vi "CallNode_Create.vi"(0 "reference":refnum<class "CallNode.lvclass">, 5 "error in (no error)":errorcluster) -> (14 "reference out":refnum<class "CallNode.lvclass">, 19 "error out":errorcluster)   [LabVIEW 2014, in "CallNode.lvclass"]
doc: "Creates and initializes a new CallNode object.\n\nThis object should be destroyed using a CallNode destructor VI or a virtual base class destructor VI.\n\n[GOOP 2.3]"
uses:
  <resource>/Framework/Providers/Open_GDS/UML/CallNode_class/CallNode.lvclass
  <resource>/Framework/Providers/Open_GDS/UML/General/Rectangle/Rectangle Rectangle2D.ctl
  <resource>/Framework/Providers/Open_GDS/UML/RectangularNode_class/RectangularNode.lvclass
panel:
  # "The input reference should only\nbe wired when this method is called\nby a sub class constructor."
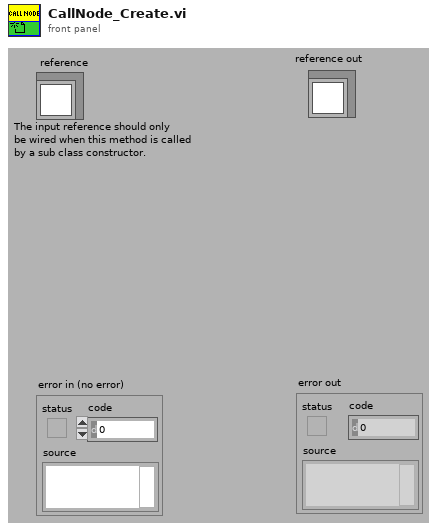
[diagram p1: front panel]
types:
  T1 = typedef "Rectangle Rectangle2D.ctl" = cluster{"x":dbl, "y":dbl, "width":dbl, "height":dbl}
  T2 = typedef "CallNode.lvclass/ClassAttributes.ctl" = cluster{"Base class":T3, "CALL_YGAP":i32}
  T3 = typedef "RectangularNode.lvclass/ClassAttributes.ctl" = cluster{"Base class":T4, "childClassAttribute2":enum16{"Hello", "Goodbye"}}
  T4 = typedef "AbstractNode.lvclass/ClassAttributes.ctl" = cluster{"classAttribute1":bool}
  T5 = typedef "CallNode.lvclass/ObjectAttributes.ctl" = cluster{"objectCallNodeRef":refnum<class "AbstractNode.lvclass">, "signaled":bool, "openBottom":bool, "DEFAULT_WIDTH":i32, "DEFAULT_HEIGHT":i32, "CALL_YGAP":i32}
  T6 = typedef "RectangularNode.lvclass/ObjectAttributes.ctl" = cluster{"bounds":T1}
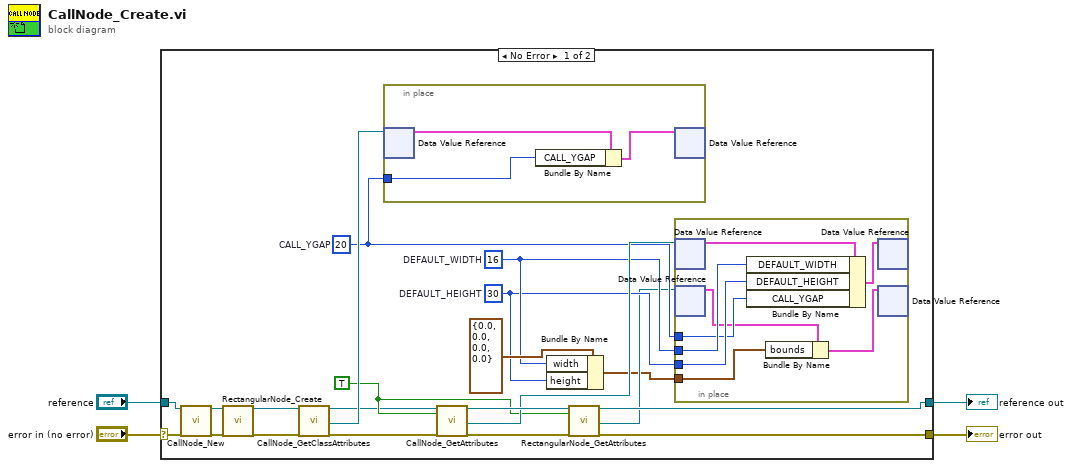
[diagram p0: block diagram]
diagram:
  n1 = case shown="No Error" "error in (no error)" {
    selector: "error in (no error)" -> [w25 w38]
    tunnel: [w12 w37] -> w4
    tunnel: [w5 w38] -> w3
    tunnel: "reference" -> [w24 w37]
    frame No Error {
      w10 = TRUE ("OnlyGetDvrReference(False)")
      w13 = 20  # CALL_YGAP
      w14 = 30  # DEFAULT_HEIGHT
      w15 = 16  # DEFAULT_WIDTH
      n2 = call <resource>:"CallNode_New.vi"("reference in"=w24, "error in (no error)"=w25) -> ("reference out"=w22:refnum<class "CallNode.lvclass">, "error out"=w23:errorcluster)  [unwired: 2 in, 14 out]
      n3 = call <resource>:"RectangularNode_Create.vi"("reference"=w22, "error in (no error)"=w23) -> ("reference out"=w19:refnum<class "CallNode.lvclass">, "error out"=w18:errorcluster)  [unwired: 1 in, 15 out]
      n4 = call <resource>:"CallNode_GetClassAttributes.vi"("reference in"=w19, "error in (no error)"=w18) -> ("reference out"=w6:refnum<class "CallNode.lvclass">, "Class attribute Reference"=w17:refnum<data-value>, "error out"=w7:errorcluster)  [unwired: 14 in, 1 out]
      n5 = in-place {
        in-place-border: w13 -> [w35]
        n6 = in-place-dvr #1(w17) -> (w36:T2)  [unwired: 1 out]
        n7 = Bundle By Name(cluster=w36, "CALL_YGAP"=w35) -> (w34:T2)
        n8 = in-place-dvr #1(w34) -> ()  [unwired: 2 out]
      }
      n9 = call <resource>:"CallNode_GetAttributes.vi"("reference in"=w6, "OnlyGetDvrReference(False)"=w10, "error in (no error)"=w7) -> ("reference out"=w21:refnum<class "CallNode.lvclass">, "DataRef"=w16:refnum<data-value>, "error out"=w11:errorcluster)  [unwired: 13 in, 1 out]
      n10 = Bundle By Name(cluster=T1 {"x"=0.0, "y"=0.0, "width"=0.0, "height"=0.0} ("Base class.bounds"), "width"=w15, "height"=w14) -> (w8:T1)
      n11 = call <resource>:"RectangularNode_GetAttributes.vi"("reference in"=w21, "OnlyGetDvrReference(False)"=w10, "error in (no error)"=w11) -> ("reference out"=w12:refnum<class "CallNode.lvclass">, "DataRef"=w9:refnum<data-value>, "error out"=w5:errorcluster)  [unwired: 13 in, 1 out]
      n12 = in-place {
        in-place-border: w15 -> [w32]
        in-place-border: w14 -> [w31]
        in-place-border: w13 -> [w30]
        in-place-border: w8 -> [w27]
        n13 = in-place-dvr #2(w16) -> (w33:T5)  [unwired: 1 out]
        n14 = in-place-dvr #3(w9) -> (w28:T6)  [unwired: 1 out]
        n15 = Bundle By Name(cluster=w33, "DEFAULT_WIDTH"=w32, "DEFAULT_HEIGHT"=w31, "CALL_YGAP"=w30) -> (w29:T5)
        n16 = Bundle By Name(cluster=w28, "bounds"=w27) -> (w26:T6)
        n17 = in-place-dvr #2(w29) -> ()  [unwired: 2 out]
        n18 = in-place-dvr #3(w26) -> ()  [unwired: 2 out]
      }
    }
    frame Error {
    }
  }
  "error out" <- w3
  "reference out" <- w4
